vi "Check Sim Controls.vi"(8 "error in (no error)":errorcluster, 11 "Simulation Controls":T1 {"Water Pressure Sensor (%)" scale=0.0..100.0}) -> (0 "error out":errorcluster, 3 "State":string)   [LabVIEW 2016]
doc: "This VI checks to see whether the pressure is below 50% or rain is present and sets the appropraite next state."
panel:
  # "Rain"
  # "No Rain"
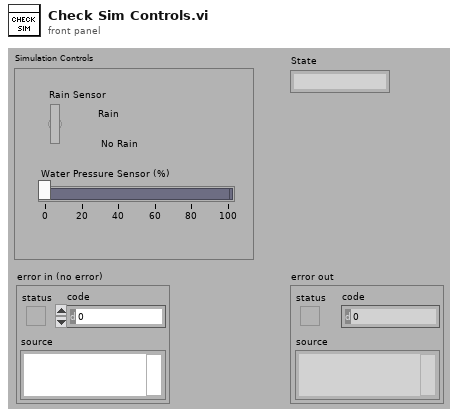
[diagram p1: front panel]
types:
  T1 = cluster{"Rain Sensor":bool, "Water Pressure Sensor (%)":dbl}
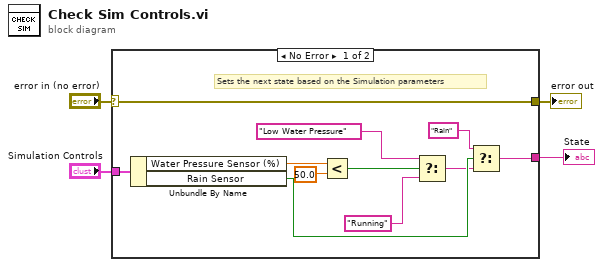
[diagram p0: block diagram]
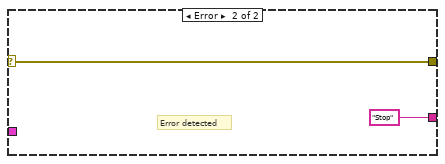
[diagram p2: hidden frame]
diagram:
  n1 = case shown="No Error" "error in (no error)" {
    selector: "error in (no error)" -> [w15 w17]
    tunnel: [w15 w17] -> w3
    tunnel: [w8 "Stop"] -> w1
    tunnel: "Simulation Controls" -> [w14 _]
    frame No Error {
      # "Sets the next state based on the Simulation parameters"
      n2 = Unbundle By Name(w14) -> ("Water Pressure Sensor (%)"=w12:dbl, "Rain Sensor"=w13:bool)
      n3 = Less?(x=w12, y=50.0) -> (x < y?=w10:bool)
      n4 = Select(t="Low Water Pressure", s=w10, f="Running") -> (s? t:f=w9:string)
      n5 = Select(t="Rain", s=w13, f=w9) -> (s? t:f=w8:string)
    }
    frame Error {
      # "Error detected"
    }
  }
  "error out" <- w3
  "State" <- w1
